vi "CMI LiB Bias Close.vi"(8 "error in":errorcluster, 11 "VISA in":refnum<visa-resource-name>) -> (0 "error out":errorcluster, 3 "VISA out":refnum<visa-resource-name>)   [LabVIEW 2013]
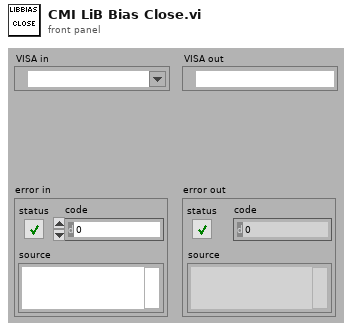
[diagram p1: front panel]
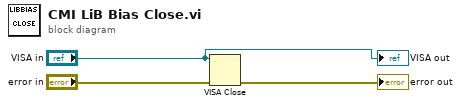
[diagram p0: block diagram]
diagram:
  n1 = VISA Close(VISA resource name="VISA in", error in (no error)="error in") -> (error out=→"error out":errorcluster)
  "VISA out" <- "VISA in"
